vi "Main.vi"(8 "error in":errorcluster, 11 "TCP Read in":refnum<class "DS TCP Read.lvclass">) -> (0 "error out":errorcluster, 3 "TCP Read out":refnum<class "DS TCP Read.lvclass">)   [LabVIEW 2017, in "DS TCP Server.lvlib" / "DS TCP Read.lvclass"]
doc: "The <b>Queued Message Handler</b> of the Worker that owns this VI."
uses:
  DS TCP Read.lvclass
  C:/Program Files (x86)/National Instruments/LabVIEW 2017/vi.lib/addons/_Workers/Library/Classes/Worker/Worker.lvclass
  Initialization Data.ctl
  <vilib>/addons/_Workers/Library/Classes/Message Queue/Message Queue.lvclass
  Response Cases.ctl
  <vilib>/addons/_Workers/Library/Case Label.ctl
  DS TCP Read.lvclass/DS TCP Read.ctl
  <vilib>/addons/_Workers/Library/Classes/Worker/Worker.lvclass/Worker.ctl
  <vilib>/addons/_Workers/Library/Classes/Message/Message.lvclass/Message.ctl
  <vilib>/addons/_Workers/Library/Classes/Message Queue/Message Queue.lvclass/Message Queue.ctl
  rsp_Connection Lost.ctl
  <vilib>/addons/_Workers/Library/Classes/Message/Enqueue Message.vi
  <vilib>/addons/_Workers/Library/Classes/Message/Bundle Standard Message.vi
  <vilib>/addons/_Workers/Library/Classes/Message Queue/Read WID.vi
  <vilib>/addons/_Workers/Library/Classes/Message/Write Priority.vi
  <vilib>/addons/_Workers/Library/Classes/Message/Write Send Message to Debugger.vi
  <vilib>/addons/_Workers/Library/Classes/Message Queue/Enqueue Element.vi
  <vilib>/addons/_Workers/Library/Classes/Message/Write Time Stamp.vi
  <vilib>/addons/_Workers/Library/Classes/Message/Write Sender WID.vi
  <vilib>/addons/_Workers/Library/Classes/Message/Write Data.vi
  <vilib>/addons/_Workers/Library/Classes/Message/Write Recipient Case.vi
  <vilib>/addons/_Workers/Library/Classes/Message/Message Time Stamp.vi
  <vilib>/addons/_Workers/Library/Classes/Message/Write Sender Case.vi
  <vilib>/addons/_Workers/Library/Classes/Worker/Read Message.vi
  <vilib>/addons/_Workers/Library/Classes/Message/Read Recipient Case.vi
  <vilib>/addons/_Workers/Library/Classes/Message/Write Auxiliary.vi
  <vilib>/addons/_Workers/Library/Classes/Worker/Read WID.vi
  <vilib>/Utility/High Resolution Relative Seconds.vi
  <vilib>/addons/_Workers/Library/Classes/Message Queue/Not a Refnum.vi
  <vilib>/Utility/error.llb/Error Cluster From Error Code.vi
  <vilib>/addons/_Workers/Library/Classes/Message/Message.lvclass
  <vilib>/addons/_Workers/Library/Workers.lvlib
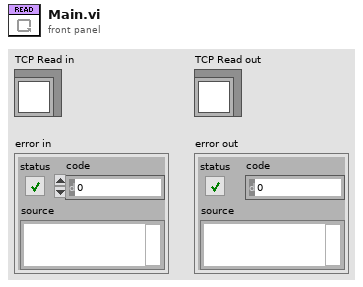
[diagram p1: front panel]
types:
  T1 = typedef "DS TCP Server.lvlib/DS TCP Read.lvclass/Initialization Data.ctl" = cluster{"Connection ID":refnum<k5>, "Forwarding Queue":refnum<class "Message Queue.lvclass">, "Response Cases":T2}
  T2 = typedef "DS TCP Server.lvlib/DS TCP Read.lvclass/Response Cases.ctl" = cluster{"Connection Lost":T3}
  T3 = typedef "Workers.lvlib/Case Label.ctl" = string
  T4 = enum16{"Standard", "Buffered", "CRLF", "Immediate"}
  T5 = cluster{"Case Label":string, "data string":string}
  T6 = typedef "DS TCP Server.lvlib/DS TCP Read.lvclass/rsp_Connection Lost.ctl" = cluster{"connection ID out":refnum<k5>, "Message Queue":refnum<class "Message Queue.lvclass">}
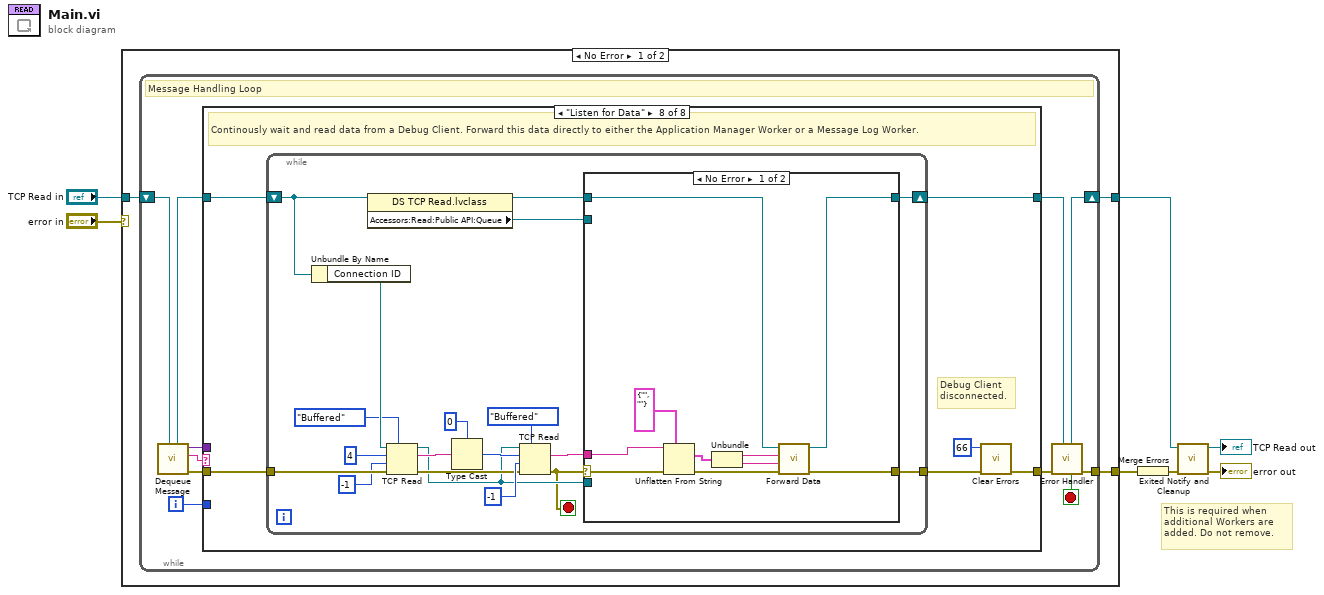
[diagram p0: block diagram]
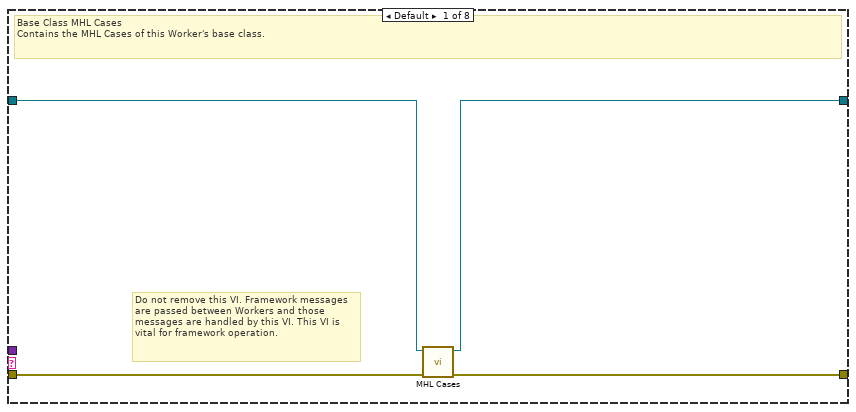
[diagram p2: hidden frame]
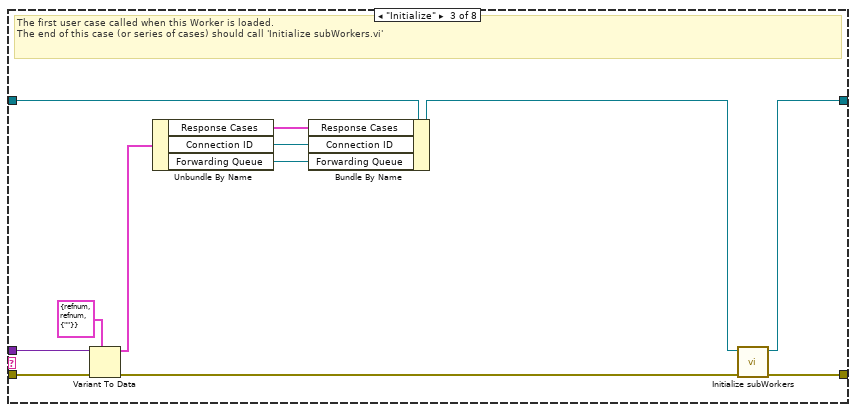
[diagram p4: hidden frame]
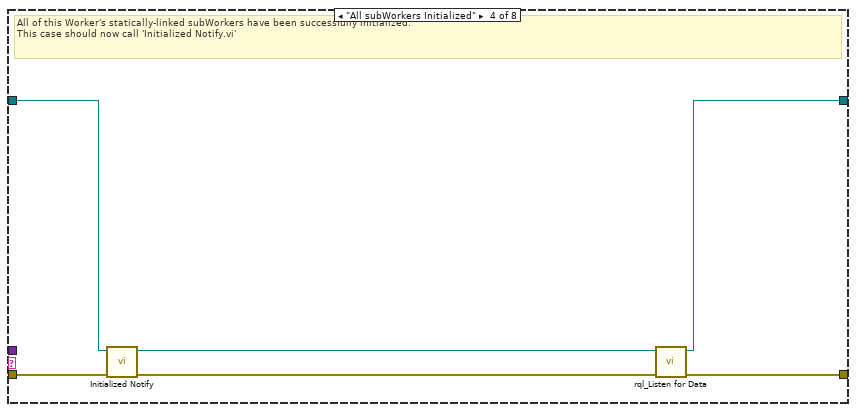
[diagram p5: hidden frame]
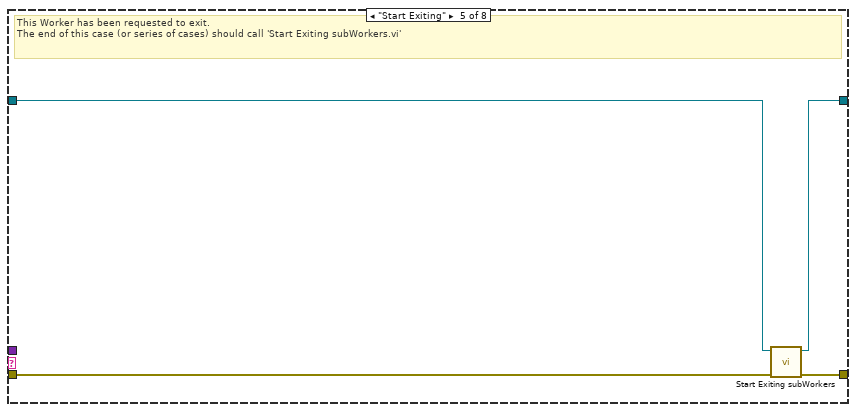
[diagram p6: hidden frame]
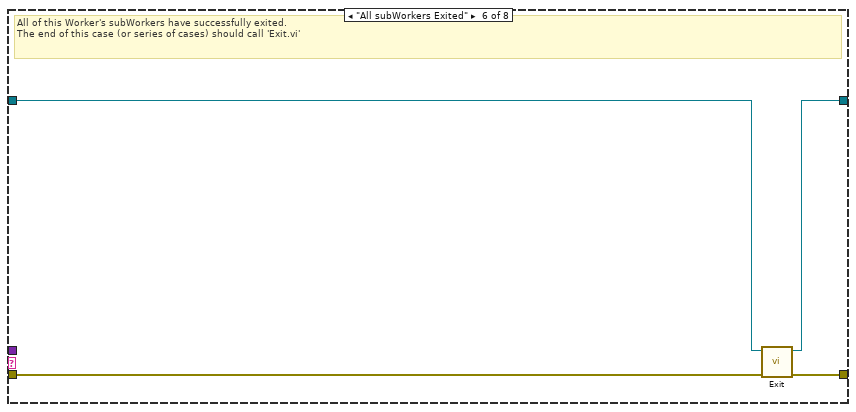
[diagram p7: hidden frame]
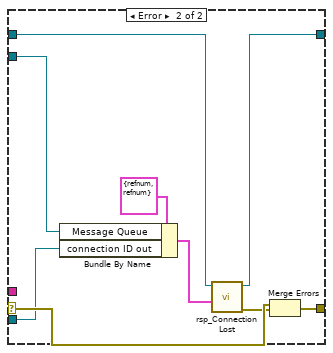
[diagram p9: hidden frame]
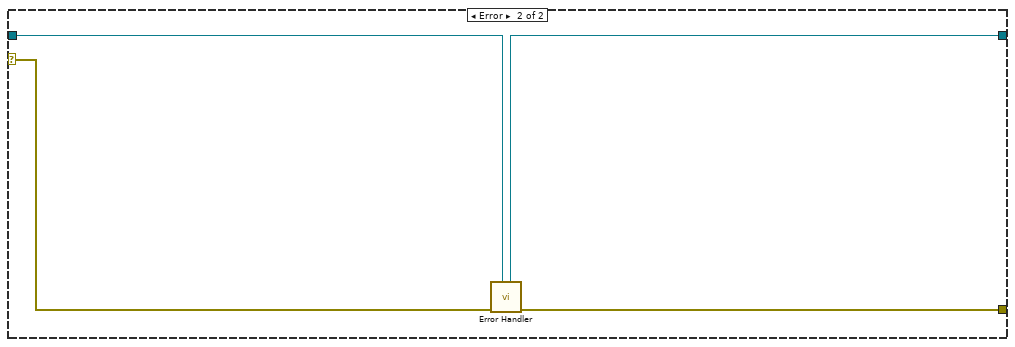
[diagram p10: hidden frame]
diagram:
  # "This is required when additional Workers are added. Do not remove."
  n1 = case shown="No Error" "error in" {
    tunnel: "TCP Read in" -> [w8 w101]
    tunnel: [w10 w102] -> w6
    tunnel: [w9 w100] -> w7
    selector: "error in" -> [_ w103]
    frame No Error {
      n2 = while {
        shift-right: [w19] -> w9
        shift-left: w8 -> [w21]
        tunnel: [w20] -> w10
        i -> [w12]
        stop <- w13 stop-if-true
        # "Message Handling Loop"
        n3 = call-dynamic "Dequeue Message.vi"("Worker"=w21) -> ("error out"=w18:errorcluster, "Case out"=w14:string, "Data out"=w11:variant, "Worker out"=w16:refnum<class "DS TCP Read.lvclass">)  [unwired: 6 in, 1 out]
        n4 = case "Worker MHL Case Structure (DO NOT CHANGE LABEL NAME)" shown="\"Listen for Data\"" w14 {
          tunnel: w18 -> [w25 w26 w37 w45 w46 w53 w55 w61]
          tunnel: [w24 w26 w39 w41 w49 w52 w55 w57] -> w17
          tunnel: w16 -> [w23 w27 w36 w43 w47 w51 w54 w60]
          tunnel: [w22 w27 w38 w40 w48 w50 w54 w59] -> w15
          tunnel: w12 -> [_ _ _ _ _ _ _ _]
          tunnel: w11 -> [_ _ w34 _ _ _ _ _]
          frame Default {
            # "Do not remove this VI. Framework messages are passed between Workers and those messages are handled by this VI. This VI is vital for framework operation."
            # "Base Class MHL Cases\nContains the MHL Cases of this Worker's base class."
            n5 = call-dynamic "MHL Cases.vi"("error in"=w25, "Worker in"=w23) -> ("error out"=w24:errorcluster, "Worker out"=w22:refnum<class "DS TCP Read.lvclass">)  [unwired: 8 in]
          }
          frame "------------ FRAMEWORK CASES -----------" {
            # "Start of Workers Framework Cases"
          }
          frame "Initialize" {
            # "The first user case called when this Worker is loaded.\nThe end of this case (or series of cases) should call 'Initialize subWorkers.vi'"
            n6 = Variant To Data(error in=w37, type=T1 {"Connection ID"=refnum, "Forwarding Queue"=refnum, "Response Cases"={"Connection Lost"=""}} ("Cluster"), Variant=w34) -> (data=w31:T1, error out=w35:errorcluster)
            n7 = Unbundle By Name(w31) -> ("Response Cases"=w28:T2, "Connection ID"=w30:refnum<k5>, "Forwarding Queue"=w29:refnum<class "Message Queue.lvclass">)
            n8 = Bundle By Name(cluster=w36, "Response Cases"=w28, "Connection ID"=w30, "Forwarding Queue"=w29) -> (w33:refnum<class "DS TCP Read.lvclass">)
            n9 = call-dynamic "Initialize subWorkers.vi"("error in"=w35, "Worker"=w33) -> ("error out"=w39:errorcluster, "dup Worker out"=w38:refnum<class "DS TCP Read.lvclass">)  [unwired: 8 in]
          }
          frame "All subWorkers Initialized" {
            # "All of this Worker's statically-linked subWorkers have been successfully initialized.\nThis case should now call 'Initialized Notify.vi'"
            n10 = call-dynamic "Initialized Notify.vi"("error in"=w45, "Worker"=w43) -> ("error out"=w44:errorcluster, "dup Worker out"=w42:refnum<class "DS TCP Read.lvclass">)  [unwired: 8 in]
            n11 = call "rql_Listen for Data.vi"("error in"=w44, "DS TCP Read in"=w42) -> ("error out"=w41:errorcluster, "dup DS TCP Read out"=w40:refnum<class "DS TCP Read.lvclass">)  [unwired: 8 in]
          }
          frame "Start Exiting" {
            # "This Worker has been requested to exit. \nThe end of this case (or series of cases) should call 'Start Exiting subWorkers.vi'"
            n12 = call-dynamic "Start Exiting subWorkers.vi"("error_in"=w46, "Worker"=w47) -> ("error out"=w49:errorcluster, "dup Worker out"=w48:refnum<class "DS TCP Read.lvclass">)  [unwired: 8 in]
          }
          frame "All subWorkers Exited" {
            # "All of this Worker's subWorkers have successfully exited. \nThe end of this case (or series of cases) should call 'Exit.vi'"
            n13 = call-dynamic "Exit.vi"("error_in"=w53, "Worker"=w51) -> ("error out"=w52:errorcluster, "dup Worker out"=w50:refnum<class "DS TCP Read.lvclass">)  [unwired: 8 in]
          }
          frame "------------- LOCAL API CASES -------------" {
            # "Start of Local API Cases"
          }
          frame "Listen for Data" {
            # "Debug Client\ndisconnected."
            # "Continously wait and read data from a Debug Client. Forward this data directly to either the Application Manager Worker or a Message Log Worker."
            n14 = while {
              shift-right: [w73] -> w59
              shift-left: w60 -> [w74]
              tunnel: w61 -> [w78]
              tunnel: [w75] -> w58
              stop <- w64 stop-if-true
              n15 = Unbundle By Name(w74) -> ("Connection ID"=w80:refnum<k5>)
              n16 = property class="DS TCP Read.lvclass"(reference=w74) -> (reference out=w63:refnum<class "DS TCP Read.lvclass">, "Accessors:Read:Public API:Queue"=w62:refnum<class "Message Queue.lvclass">)  [unwired: 1 in, 1 out]
              n17 = TCP Read(connection ID=w80, bytes to read=4, error in (no error)=w78, 7:T4."Buffered" ("mode (standard)"), 9:-1 ("timeout ms (25000)")) -> (connection ID out=w66:refnum<k5>, data out=w67:string, error out=w68:errorcluster)
              n18 = Type Cast(type=0 ("bytes to read"), x=w67) -> (*(type *) &x=w70:i32)
              n19 = TCP Read(connection ID=w66, bytes to read=w70, error in (no error)=w68, 7:T4."Buffered" ("mode (standard)"), 9:-1 ("timeout ms (25000)")) -> (data out=w65:string, error out=w64:errorcluster)  [unwired: 1 out]
              n20 = case shown="No Error" w64 {
                selector: w64 -> [w87 w96]
                tunnel: [w84 w99] -> w75
                tunnel: w66 -> [_ w91]
                tunnel: w63 -> [w90 w98]
                tunnel: [w83 w97] -> w73
                tunnel: w65 -> [w86 _]
                tunnel: w62 -> [_ w92]
                frame No Error {
                  n21 = Unflatten From String(type=T5 {"Case Label"="", "data string"=""} ("element"), binary string=w86, error in (no error)=w87) -> (value=w89:T5, error out=w88:errorcluster)  [unwired: 2 in, 1 out]
                  n22 = Unbundle(w89) -> ("Case Label"=w81:string, "data string"=w82:string)
                  n23 = call "Forward Data.vi"("error in (no error)"=w88, "Data"=w82, "Forwarding Case"=w81, "TCP Read in"=w90) -> ("error out"=w84:errorcluster, "TCP Read out"=w83:refnum<class "DS TCP Read.lvclass">)  [unwired: 6 in]
                }
                frame Error {
                  n24 = Bundle By Name(cluster=T6 {"connection ID out"=refnum, "Message Queue"=refnum} ("Data in"), "Message Queue"=w92, "connection ID out"=w91) -> (w93:T6)
                  n25 = call "rsp_Connection Lost.vi"("Data in"=w93, "DS TCP Read in"=w98) -> ("error out"=w95:errorcluster, "dup DS TCP Read out"=w97:refnum<class "DS TCP Read.lvclass">)  [unwired: 8 in]
                  n26 = Merge Errors(w96, w95) -> (w99:errorcluster)
                }
              }
            }
            n27 = call <vilib>:"Clear Errors.vi"("error in (no error)"=w58, "specific error code to clear (0: all)"=66) -> ("error out"=w57:errorcluster)  [unwired: 4 in, 1 out]
          }
        }
        n28 = call-dynamic "Error Handler.vi"("Worker"=w15, "error_in"=w17) -> ("error out"=w20:errorcluster, "Stop Loop"=w13:bool, "Worker out"=w19:refnum<class "DS TCP Read.lvclass">)  [unwired: 7 in]
      }
    }
    frame Error {
      n29 = call-dynamic "Error Handler.vi"("Worker"=w101, "error_in"=w103) -> ("error out"=w102:errorcluster, "Worker out"=w100:refnum<class "DS TCP Read.lvclass">)  [unwired: 7 in, 1 out]
    }
  }
  n30 = Merge Errors(w6) -> (w3:errorcluster)
  n31 = call-dynamic "Exited Notify and Cleanup.vi"("error_in"=w3, "Worker"=w7) -> ("error out"=→"error out":errorcluster, "dup Worker out"=→"TCP Read out":refnum<class "DS TCP Read.lvclass">)  [unwired: 8 in]
